vi "Event Create.vi"(9 "Event Actor":refnum<class "Event Actor.lvclass">, 10 "Alias":string, 11 "Event Create in":refnum<class "Event Create.lvclass">) -> (3 "Event Create out":refnum<class "Event Create.lvclass">)   [LabVIEW 2021, in "jettl.lvlib" / "Event Create.lvlib" / "Event Create.lvclass"]
uses:
  Event Create.lvclass
  Event Actor/Event Actor.lvclass
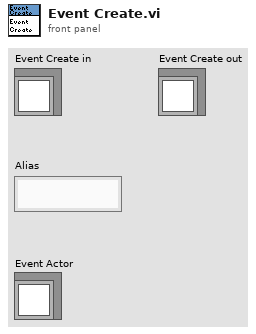
[diagram p1: front panel]
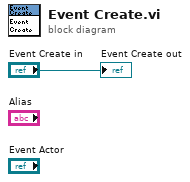
[diagram p0: block diagram]
diagram:
  "Event Create out" <- "Event Create in"
